vi "HEWH RLT PRAT Data Parse Specific Data.vi"(0 "Data (Label,Data) In":string[][](array[string])=[["Voltage (V)", "0.000"], ["RMS Current (Amps)", "0.000"], ["Power (Watts)", "0.000"], ["Watt Hours (Wh)", "0.000"], ["Voltage Total Harmonic Distortion", "0.000"], ["Frequency (Hz)", "0.000"], ["Apparent Power (VA)", "0.000"], ["Power Factor", "0.000"], ["Current Crest Factor", "0.000"], ["Voltage Crest Factor", "0.000"], ["Integration Time (sec)", "0.000"], ["Intellifaucet Valve % Open", "0.000"], ["TC Tree Average", "0.000"], ["TC Down", "0.000"], ["RTD IN", "0.000"], ["RTD Out", "0.000"], ["RTD Ambient", "0.000"], ["Totalized Flow (Linear Link) - Calculated (Gallons)", "20.50"], ["Flow Rate (Linear Link) - Calculated (GPM)", "3.00"], ["Pressure - HI1", "0.000"], ["Pressure - HI2", "0.000"], ["Pressure - LOW", "0.000"], ["Pressure - PIN", "0.000"]], 5 "Error In":errorcluster, 6 "Station ID":string="A", 7 "Current Drawing Station":string="A", 9 "Show Flow Data":bool) -> (12 "Current (Amps)":dbl, 14 "Data (Label,Data) Out":string[][](array[string])=[["Voltage (V)", "0.000"], ["RMS Current (Amps)", "0.000"], ["Power (Watts)", "0.000"], ["Watt Hours (Wh)", "0.000"], ["Voltage Total Harmonic Distortion", "0.000"], ["Frequency (Hz)", "0.000"], ["Apparent Power (VA)", "0.000"], ["Power Factor", "0.000"], ["Current Crest Factor", "0.000"], ["Voltage Crest Factor", "0.000"], ["Integration Time (sec)", "0.000"], ["Intellifaucet Valve % Open", "0.000"], ["TC Tree Average", "0.000"], ["TC Down", "0.000"], ["RTD IN", "0.000"], ["RTD Out", "0.000"], ["RTD Ambient", "0.000"], ["Totalized Flow (Linear Link) - Calculated (Gallons)", "20.50"], ["Flow Rate (Linear Link) - Calculated (GPM)", "3.00"], ["Pressure - HI1", "0.000"], ["Pressure - HI2", "0.000"], ["Pressure - LOW", "0.000"], ["Pressure - PIN", "0.000"]], 19 "Error Out":errorcluster)   [LabVIEW 2020]
uses:
  <vilib>/Utility/error.llb/whitespace.ctl
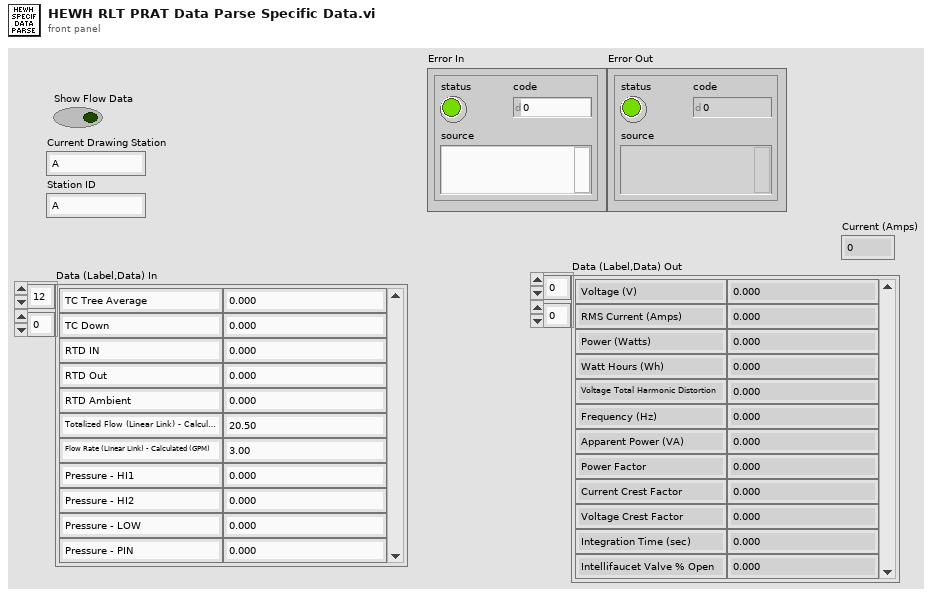
[diagram p1: front panel]
types:
  T1 = typedef "whitespace.ctl" = u16
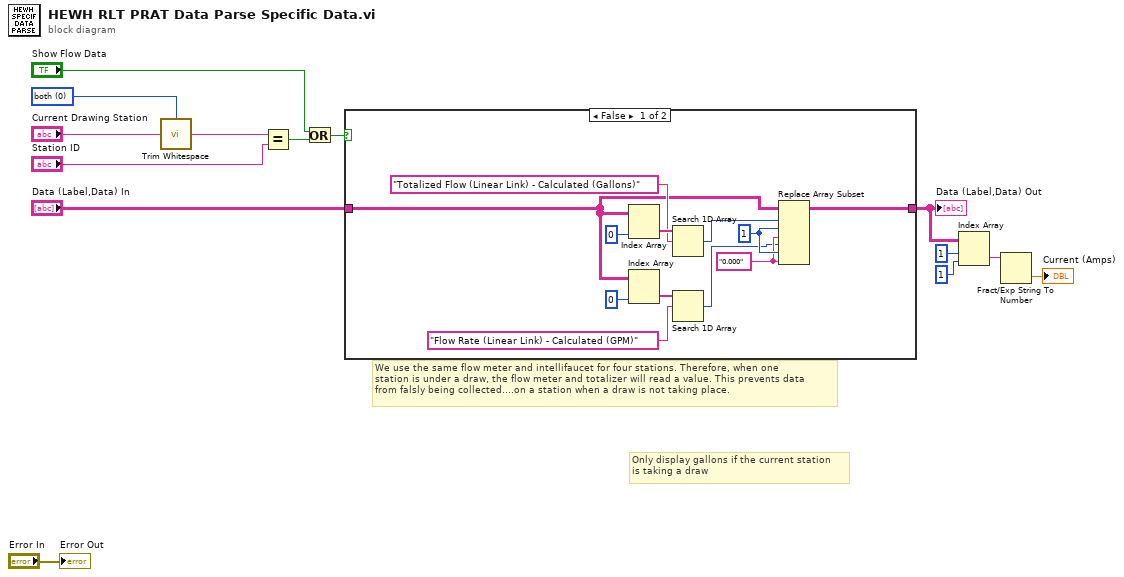
[diagram p0: block diagram]
diagram:
  w11 = T1 0 items=["both", "start of string", "end of string"] ("location (both)")
  # "We use the same flow meter and intellifaucet for four stations. Therefore, when one \nstation is under a draw, the flow meter and totalizer will read a value. This prevents data \nfrom falsly being collected....on a station when a draw is not taking place."
  # "Only display gallons if the current station\nis taking a draw"
  n1 = call <vilib>:"Trim Whitespace.vi"("string"="Current Drawing Station", "location (both)"=w11) -> ("trimmed string"=w9:string)
  n2 = Equal?(x=w9, y="Station ID") -> (x = y?=w3:bool)
  n3 = Or(x="Show Flow Data", y=w3) -> (x .or. y?=w1:bool)
  n4 = case shown="False" w1 {
    tunnel: "Data (Label,Data) In" -> [w17 w27]
    tunnel: [w24 w27] -> w8
    frame False {
      w26 = 1 ("disabled index (col)")
      w25 = "0.000" ("new element/subarray")
      n5 = Index Array(array=w17, index (col)=0 ("disabled index (col)")) -> (element=w22:string[])  [unwired: 1 in]
      n6 = Index Array(array=w17, index (col)=0 ("disabled index (col)")) -> (element=w19:string[])  [unwired: 1 in]
      n7 = Search 1D Array(1D array=w22, element="Totalized Flow (Linear Link) - Calculated (Gallons)") -> (index of element=w20:i32)  [unwired: 1 in]
      n8 = Search 1D Array(1D array=w19, element="Flow Rate (Linear Link) - Calculated (GPM)") -> (index of element=w15:i32)  [unwired: 1 in]
      n9 = Replace Array Subset(array=w17, new element #1=w25, index (row) #1=w20, index (col) #1=w26, new element #2=w25, index (row) #2=w15, index (col) #2=w26) -> (w24:string[][])
    }
    frame True {
    }
  }
  "Data (Label,Data) Out" <- w8
  n10 = Index Array(array=w8, index (row)=1 ("disabled index (row)"), index (col)=1 ("disabled index (col)")) -> (element=w5:string)
  n11 = Fract/Exp String To Number(string=w5) -> (number=→"Current (Amps)":dbl)  [unwired: 3 in, 1 out]
  "Error Out" <- "Error In"
